vi "Init3456.vi"(2 "error in (no error)":errorcluster, 3 "VISA session 2":refnum<visa-resource-name>) -> (0 "error out":errorcluster, 1 "VISA session":refnum<visa-resource-name>)   [LabVIEW 2012]
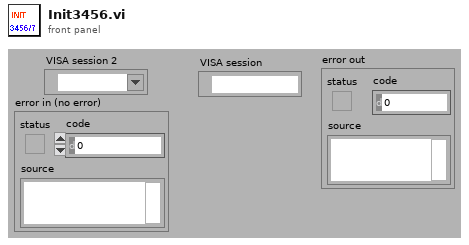
[diagram p1: front panel]
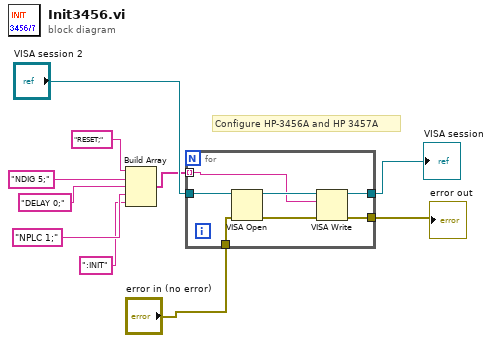
[diagram p0: block diagram]
diagram:
  # "Configure HP-3456A and HP 3457A"
  n1 = Build Array("RESET;", "NDIG 5;", "DELAY 0;", "NPLC 1;" ("element"), ":INIT" ("element")) -> (w6:string[])
  n2 = for {
    tunnel: w6 -> [w15] mode=indexing
    tunnel: "VISA session 2" -> [w17]
    tunnel: [w13] -> w9
    tunnel: [w12] -> w10
    tunnel: "error in (no error)" -> [w11]
    n3 = VISA Open(error in (no error)=w11, VISA resource name=w17) -> (VISA resource name=w16:refnum<visa-resource-name>, error out=w14:errorcluster)  [unwired: 3 in]
    n4 = VISA Write(VISA resource name=w16, write buffer=w15, error in (no error)=w14) -> (VISA resource name out=w13:refnum<visa-resource-name>, error out=w12:errorcluster)  [unwired: 1 out]
  }
  "error out" <- w10
  "VISA session" <- w9
